vi "ElevatorTeleop.vi"(0 "CmdElevAlgae2":bool, 1 "CmdElevL3":bool, 2 "CmdElevAlgae1":bool, 3 "CmdElevSource":bool, 4 "CmdElevL2":bool, 5 "CmdElevL1":bool, 6 "CmdElevL4":bool, 7 "CmdElevRest":bool, 8 "CmdBarge":bool, 9 "CmdFloor":bool, 10 "CmdElevDec":bool, 11 "CmdElevCancel":bool, 12 "CmdElevInc":bool, 13 "CmdProcessor":bool) -> ()   [LabVIEW 2023]
doc: "Makes sure the actual position of the arm is within 5 degrees of the setpoint/target"
uses:
  <vilib>/Rock Robotics/WPI/ThirdParty/JAS_Junk/TrajLib/VI/BoolCmd_Send.vi
  Wrist/WristCancelSendCmd.vi
  <vilib>/Rock Robotics/WPI/ThirdParty/JAS_Junk/TrajLib/VI/BoolCmd_Send_Internal.vi
  <vilib>/Rock Robotics/WPI/ThirdParty/JAS_Junk/TrajLib/VI/BoolCmd_ObtainQueue.vi
  <vilib>/Rock Robotics/WPI/ThirdParty/JAS_Junk/TrajLib/Trajectory_Library.lvlib
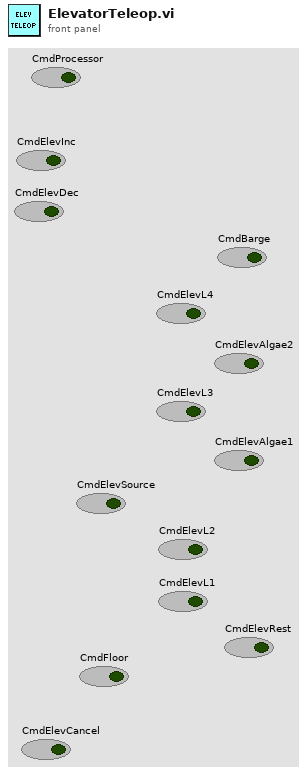
[diagram p1: front panel]
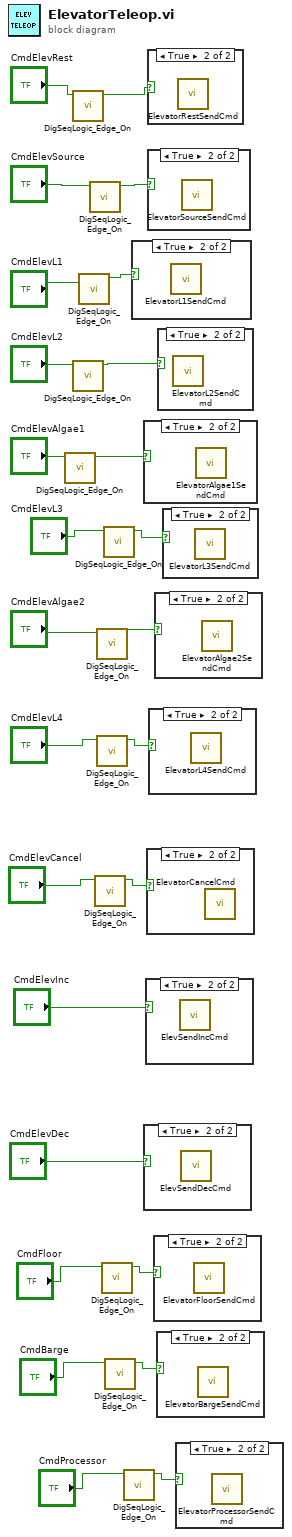
[diagram p0: block diagram]
diagram:
  n1 = call <vilib>:"DigSeqLogic_Edge_On.vi"("Input"="CmdElevAlgae1") -> ("On Edge"=w25:bool)  [unwired: 10 in]
  n2 = call <vilib>:"DigSeqLogic_Edge_On.vi"("Input"="CmdElevRest") -> ("On Edge"=w17:bool)  [unwired: 10 in]
  n3 = call <vilib>:"DigSeqLogic_Edge_On.vi"("Input"="CmdElevL2") -> ("On Edge"=w23:bool)  [unwired: 10 in]
  n4 = call <vilib>:"DigSeqLogic_Edge_On.vi"("Input"="CmdElevL1") -> ("On Edge"=w26:bool)  [unwired: 10 in]
  n5 = call <vilib>:"DigSeqLogic_Edge_On.vi"("Input"="CmdElevSource") -> ("On Edge"=w24:bool)  [unwired: 10 in]
  n6 = call <vilib>:"DigSeqLogic_Edge_On.vi"("Input"="CmdElevCancel") -> ("On Edge"=w9:bool)  [unwired: 10 in]
  n7 = call <vilib>:"DigSeqLogic_Edge_On.vi"("Input"="CmdElevAlgae2") -> ("On Edge"=w14:bool)  [unwired: 10 in]
  n8 = call <vilib>:"DigSeqLogic_Edge_On.vi"("Input"="CmdElevL4") -> ("On Edge"=w11:bool)  [unwired: 10 in]
  n9 = call <vilib>:"DigSeqLogic_Edge_On.vi"("Input"="CmdFloor") -> ("On Edge"=w8:bool)  [unwired: 10 in]
  n10 = call <vilib>:"DigSeqLogic_Edge_On.vi"("Input"="CmdElevL3") -> ("On Edge"=w15:bool)  [unwired: 10 in]
  n11 = call <vilib>:"DigSeqLogic_Edge_On.vi"("Input"="CmdBarge") -> ("On Edge"=w4:bool)  [unwired: 10 in]
  n12 = call <vilib>:"DigSeqLogic_Edge_On.vi"("Input"="CmdProcessor") -> ("On Edge"=w2:bool)  [unwired: 10 in]
  n13 = case shown="True" w26 {
    frame False {
    }
    frame True {
      n14 = call "ElevatorL1SendCmd.vi"() -> ()  [unwired: 11 in, 1 out]
    }
  }
  n15 = case shown="True" w25 {
    frame False {
    }
    frame True {
      n16 = call "ElevatorAlgae1SendCmd.vi"() -> ()  [unwired: 11 in, 1 out]
    }
  }
  n17 = case shown="True" "CmdElevDec" {
    frame False {
    }
    frame True {
      n18 = call "ElevSendDecCmd.vi"() -> ()  [unwired: 11 in, 1 out]
    }
  }
  n19 = case shown="True" "CmdElevInc" {
    frame False {
    }
    frame True {
      n20 = call "ElevSendIncCmd.vi"() -> ()  [unwired: 11 in, 1 out]
    }
  }
  n21 = case shown="True" w9 {
    frame False {
    }
    frame True {
      n22 = call "ElevatorCancelCmd.vi"() -> ()  [unwired: 11 in, 1 out]
    }
  }
  n23 = case shown="True" w17 {
    frame False {
    }
    frame True {
      n24 = call "ElevatorRestSendCmd.vi"() -> ()  [unwired: 11 in, 1 out]
    }
  }
  n25 = case shown="True" w24 {
    frame False {
    }
    frame True {
      n26 = call "ElevatorSourceSendCmd.vi"() -> ()  [unwired: 11 in, 1 out]
    }
  }
  n27 = case shown="True" w11 {
    frame False {
    }
    frame True {
      n28 = call "ElevatorL4SendCmd.vi"() -> ()  [unwired: 11 in, 1 out]
    }
  }
  n29 = case shown="True" w8 {
    frame False {
    }
    frame True {
      n30 = call "ElevatorFloorSendCmd.vi"() -> ()  [unwired: 11 in, 1 out]
    }
  }
  n31 = case shown="True" w14 {
    frame False {
    }
    frame True {
      n32 = call "ElevatorAlgae2SendCmd.vi"() -> ()  [unwired: 11 in, 1 out]
    }
  }
  n33 = case shown="True" w4 {
    frame False {
    }
    frame True {
      n34 = call "ElevatorBargeSendCmd.vi"() -> ()  [unwired: 11 in, 1 out]
    }
  }
  n35 = case shown="True" w23 {
    frame False {
    }
    frame True {
      n36 = call "ElevatorL2SendCmd.vi"() -> ()  [unwired: 11 in, 1 out]
    }
  }
  n37 = case shown="True" w15 {
    frame False {
    }
    frame True {
      n38 = call "ElevatorL3SendCmd.vi"() -> ()  [unwired: 11 in, 1 out]
    }
  }
  n39 = case shown="True" w2 {
    frame False {
    }
    frame True {
      n40 = call "ElevatorProcessorSendCmd.vi"() -> ()  [unwired: 11 in, 1 out]
    }
  }
